vi "QT_MatrixSkew.vi"(0 "In Matrix [3x3] (Identity)":dbl[][](array[numeric])=[[1.0, 0.0, 0.0], [0.0, 1.0, 0.0], [0.0, 0.0, 1.0]] format="%.2f", 7 "X skew":dbl format="%.2f", 9 "Y skew":dbl format="%.2f", 11 "error in (no error)":errorcluster) -> (4 "Out Matrix":dbl[][](array[numeric])=[[1.0, 0.0, 0.0], [0.0, 1.0, 0.0], [0.0, 0.0, 1.0]] format="%.2f", 10 "Out Matrix as Vector":dbl[](array[numeric])=[1.0, 0.0, 0.0] format="%.2f", 15 "error out":errorcluster)   [LabVIEW 2024]
uses:
  <vilib>/Analysis/baseanly.llb/Real A x B.vi
  <vilib>/Analysis/NI_AALBase.lvlib
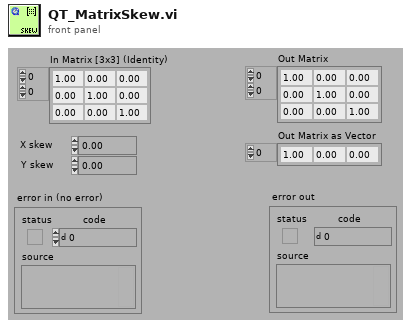
[diagram p1: front panel]
types:
  T1 = typedef "NI_Matrix.lvlib/RealMatrix.ctl" = dbl[][]
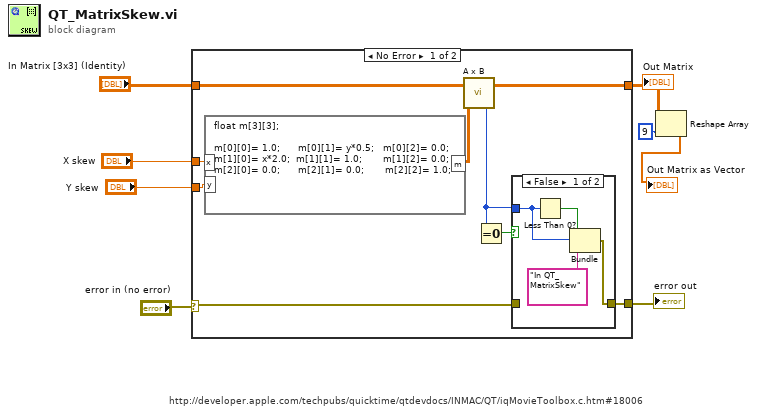
[diagram p0: block diagram]
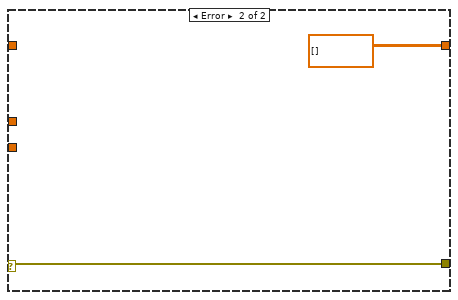
[diagram p3: hidden frame]
diagram:
  # "http://developer.apple.com/techpubs/quicktime/qtdevdocs/INMAC/QT/iqMovieToolbox.c.htm#18006"
  n1 = case shown="No Error" "error in (no error)" {
    selector: "error in (no error)" -> [w10 w23]
    tunnel: [w17 dbl[][] [] ("A x B")] -> w8
    tunnel: "In Matrix [3x3] (Identity)" -> [w16 _]
    tunnel: "X skew" -> [w14 _]
    tunnel: [w13 w23] -> w4
    tunnel: "Y skew" -> [w9 _]
    frame No Error {
      n2 = formula code="float m[3][3];\n\nm[0][0]= 1.0;      m[0][1]= y*0.5;   m[0][2]= 0.0;\nm[1][0]= x*2.0;  m[1][1]= 1.0;       m[1][2]= 0.0;\nm[2][0]= 0.0;      m[2][1]= 0.0;       m[2][2]= 1.0;"("x"=w14, "y"=w9) -> ("m"=w15:dbl[][])
      n3 = call-poly <vilib>:"A x B.vi"("B"=w15, "A"=w16) -> ("error"=w12:i32, "A x B"=w17:T1)
      n4 = Equal To 0?(x=w12) -> (x = 0?=w11:bool)
      n5 = case shown="False" w11 {
        tunnel: [w21 w22] -> w13
        tunnel: w12 -> [w19 _]
        tunnel: w10 -> [_ w22]
        frame False {
          n6 = Less Than 0?(x=w19) -> (x < 0?=w20:bool)
          n7 = Bundle(w20, "error"=w19, "In QT_MatrixSkew") -> (w21:cluster{bool, "error":i32, string})  [unwired: 1 out]
        }
        frame True {
        }
      }
    }
    frame Error {
    }
  }
  "Out Matrix" <- w8
  "error out" <- w4
  n8 = Reshape Array(w8, 9 ("dimension size")) -> (→"Out Matrix as Vector":dbl[])
